vi "Pusher_Client_UnSubscribe.vi"(8 "ErrIn":errorcluster, 10 "ChannelName":string, 11 "Client in":refnum<class "Client.lvclass">) -> (0 "ErrOut":errorcluster, 3 "Client out":refnum<class "Client.lvclass">)   [LabVIEW 2009, in "Client.lvclass"]
uses:
  Client.lvclass
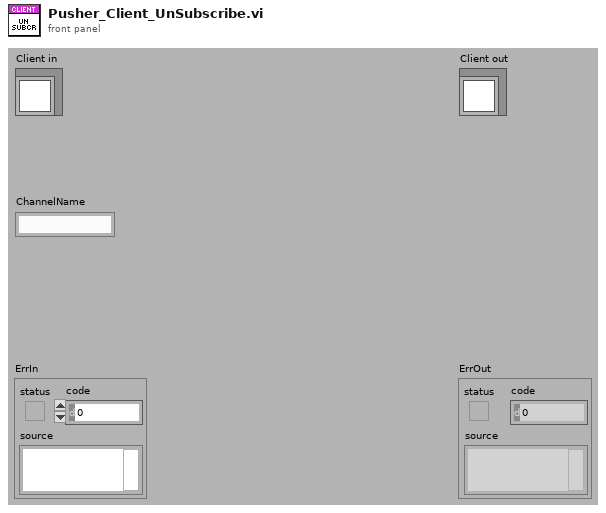
[diagram p1: front panel]
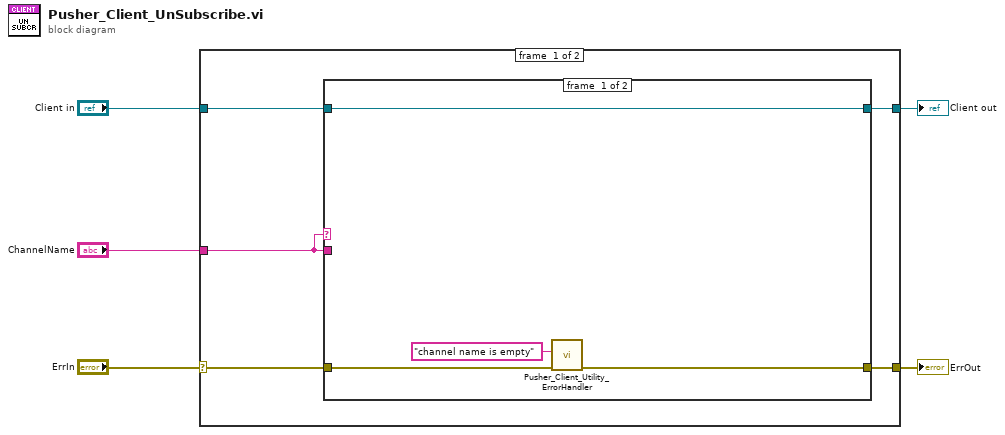
[diagram p0: block diagram]
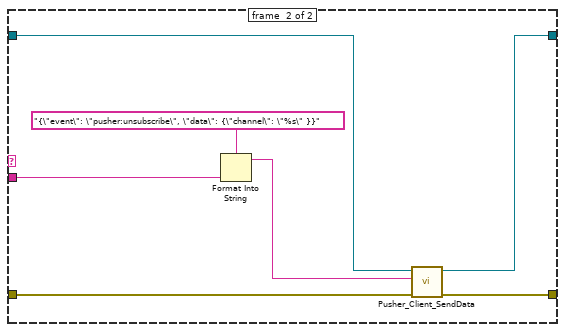
[diagram p2: hidden frame]
diagram:
  n1 = case shown="No Error" "ErrIn" {
    selector: "ErrIn" -> [w10 w23]
    tunnel: [w9 w23] -> w4
    tunnel: [w7 w22] -> w2
    tunnel: "Client in" -> [w8 w22]
    tunnel: "ChannelName" -> [w6 _]
    frame #0 {
      n2 = case shown="\"True\", Default" w6 {
        tunnel: w10 -> [w13 w21]
        tunnel: [w12 w20] -> w9
        tunnel: w8 -> [w14 w19]
        tunnel: [w14 w18] -> w7
        tunnel: w6 -> [_ w17]
        frame #0 {
          n3 = call "Pusher_Client_Utility_ErrorHandler.vi"("ErrIn"=w13, "Additional Message"="channel name is empty") -> ("ErrOut"=w12:errorcluster)  [unwired: 9 in]
        }
        frame #1 {
          n4 = Format Into String(format string="{\"event\": \"pusher:unsubscribe\", \"data\": {\"channel\": \"%s\" }}", w17) -> (resulting string=w15:string)  [unwired: 2 in, 1 out]
          n5 = call "Pusher_Client_SendData.vi"("ErrIn"=w21, "data"=w15, "Client in"=w19) -> ("ErrOut"=w20:errorcluster, "Client out"=w18:refnum<class "Client.lvclass">)  [unwired: 7 in]
        }
      }
    }
    frame #1 {
    }
  }
  "ErrOut" <- w4
  "Client out" <- w2
